vi "Return_Specific_Header.vi"(8 "error in (no error)":errorcluster, 10 "Specific Header":string, 11 "Response in":refnum<class "Response.lvclass">) -> (0 "error out":errorcluster, 2 "Specific Header":string[](array[string]), 3 "Response out":refnum<class "Response.lvclass">)   [LabVIEW 2016, in "Response.lvclass"]
uses:
  Response.lvclass
  Response.lvclass/Response.ctl
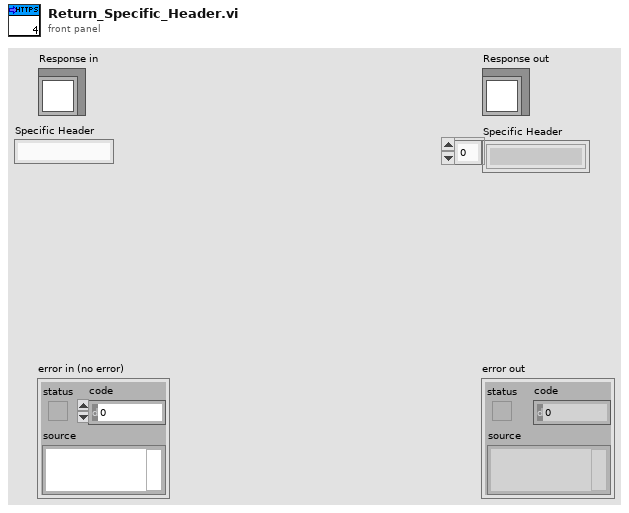
[diagram p1: front panel]
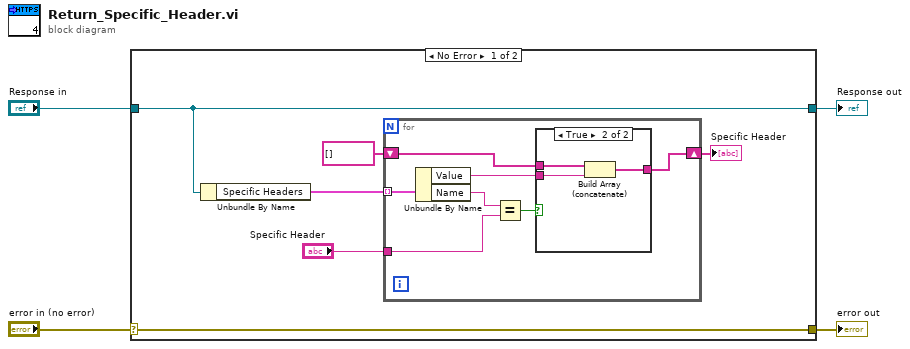
[diagram p0: block diagram]
diagram:
  n1 = case shown="No Error" "error in (no error)" {
    selector: "error in (no error)" -> [w10 w23]
    tunnel: [w10 w23] -> w3
    tunnel: [w9 w22] -> w1
    tunnel: "Response in" -> [w9 w22]
    frame No Error {
      n2 = Unbundle By Name(w9) -> ("Specific Headers"=w8:cluster{"Name":string, "Value":string}[])
      n3 = for {
        tunnel: w8 -> [w17] mode=indexing
        tunnel: "Specific Header" -> [w15]
        shift-right: [w12] -> w5
        shift-left: string[] [] -> [w11]
        n4 = Unbundle By Name(w17) -> ("Value"=w13:string, "Name"=w16:string)
        n5 = Equal?(x=w16, y=w15) -> (x = y?=w14:bool)
        n6 = case shown="True" w14 {
          tunnel: w13 -> [_ w21]
          tunnel: [w18 w20] -> w12
          tunnel: w11 -> [w18 w19]
          frame False {
          }
          frame True {
            n7 = Build Array (concatenate)(w19, w21) -> (w20:string[])
          }
        }
      }
      "Specific Header" <- w5
    }
    frame Error {
    }
  }
  "error out" <- w3
  "Response out" <- w1
